vi "ExCenterStripStrNframe.vi"() -> ()   [LabVIEW 2010]
panel:
  in  "Number of frames to store":u32=1 min=1 step=1
  out "Strip":sgl[](graph)
  in  "Temperature":dbl=-10.0 format="%.2f"
  in  "Exposure":dbl min=0.0 step=0.001 format="%.3f"
  out "error out":errorcluster
  in  "error in (no error)":errorcluster
  # "ExCenterStripStrNframe:\nThis example selects the center strip of the CCD for the ROI and then \ncollects the data using circular buffers. It collects data until the number \nof frames are stored."
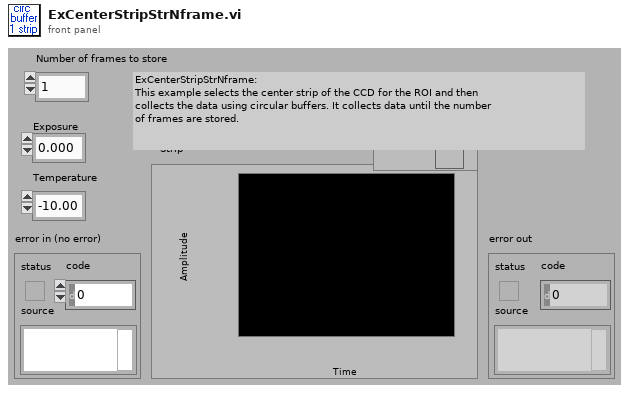
[diagram p1: front panel]
types:
  T1 = cluster{"Acquire / focus mode \n1 is Sync circualar buffers":i32, "Exposure":dbl, "Number of frames to store":u32, "Number of software\naccumulations":i32}
  T2 = cluster{"Camera Handle":u32, "Pulser Handle":u32, "File Handle":u32, "Display Handle":u32, "Image Handle":u32}
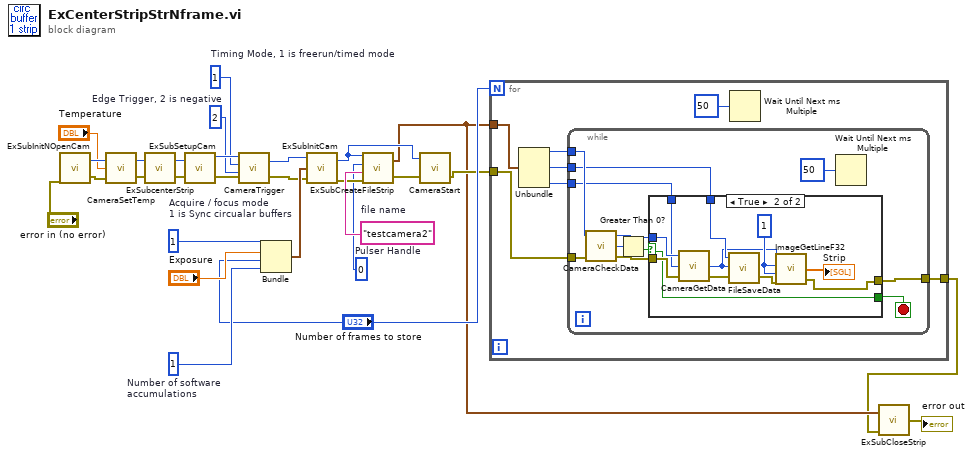
[diagram p0: block diagram]
diagram:
  w14 = 2  # Edge Trigger, 2 is negative
  w15 = 1  # Timing Mode, 1 is freerun/timed mode
  w21 = 0  # Pulser Handle
  w27 = 1  # Acquire / focus mode  1 is Sync circualar buffers
  w26 = 1  # Number of software accumulations
  w28 = "testcamera2"  # file name
  n1 = call "ExSubInitNOpenCam.vi"("error in (no error)"="error in (no error)") -> ("Camera Handle"=w7:u32, "error out"=w6:errorcluster)
  n2 = call <userlib>:"CameraSetTemp.vi"("error in (no error)"=w6, "Temperature"="Temperature", "Camera Handle"=w7) -> ("error out"=w8:errorcluster, "Camera Handle"=w9:u32)
  n3 = call "ExSubcenterStrip.vi"("error in (no error)"=w8, "Camera Handle"=w9) -> ("error out"=w11:errorcluster, "Camera Handle"=w10:u32)
  n4 = call "ExSubSetupCam.vi"("error in (no error)"=w11, "Camera Handle"=w10) -> ("error out"=w13:errorcluster, "Camera Handle"=w17:u32)
  n5 = call <userlib>:"CameraTrigger.vi"("error in"=w13, "Trigger Edge"=w14, "Timing Mode"=w15, "Camera Handle"=w17) -> ("error out"=w18:errorcluster, "Camera Handle"=w16:u32)
  n6 = Bundle("Acquire / focus mode \n1 is Sync circualar buffers"=w27, "Exposure"="Exposure", "Number of frames to store"="Number of frames to store", "Number of software\naccumulations"=w26) -> (w23:T1)  [unwired: 1 in]
  n7 = call "ExSubInitCam.vi"("error in (no error)"=w18, "Camera Information"=w23, "Camera Handle"=w16) -> ("error out"=w22:errorcluster, "Camera Handle"=w20:u32)
  n8 = call "ExSubCreateFileStrip.vi"("error in (no error)"=w22, "File and Display Name"=w28, "Pulser Handle"=w21, "Camera Handle"=w20) -> ("error out"=w12:errorcluster, "Handles Out"=w2:T2)
  n9 = call <userlib>:"CameraStart.vi"("error in"=w12, "Camera Handle"=w20) -> ("error out"=w3:errorcluster)  [unwired: 1 out]
  n10 = for {
    N: "Number of frames to store" -> [_]
    tunnel: w2 -> [w35]
    tunnel: w3 -> [w30]
    tunnel: [w29] -> w1
    n11 = Unbundle(w35) -> ("Camera Handle"=w34:u32, "File Handle"=w32:u32, "Image Handle"=w33:u32)  [unwired: 2 out]
    n12 = while {
      tunnel: [w41] -> w29
      tunnel: w34 -> [w39]
      tunnel: w33 -> [w38]
      tunnel: w32 -> [w37]
      tunnel: w30 -> [w36]
      stop <- w42 stop-if-true
      n13 = call <userlib>:"CameraCheckData.vi"("Camera Handle"=w39, "error in"=w36) -> ("Camera Handle"=w44:u32, "Number Of Frames Available"=w46:i32, "error out"=w43:errorcluster)
      n14 = Greater Than 0?(x=w46) -> (x > 0?=w45:bool)
      n15 = case shown="True" w45 {
        selector: w45 -> [w47 w57]
        tunnel: w44 -> [_ w59]
        tunnel: w43 -> [w48 w58]
        tunnel: [w47 w57] -> w42
        tunnel: [w48 w52] -> w41
        tunnel: w38 -> [_ w51]
        tunnel: w37 -> [_ w50]
        frame False {
        }
        frame True {
          w53 = 1
          n16 = call <userlib>:"CameraGetData.vi"("error in"=w58, "Data Handle"=w51, "Camera Handle"=w59) -> ("error out"=w56:errorcluster, "Data Handle"=w49:u32)  [unwired: 1 out]
          n17 = call <userlib>:"FileSaveData.vi"("error in"=w56, "Image Handle"=w49, "File Handle"=w50) -> ("error out"=w55:errorcluster)  [unwired: 1 out]
          n18 = call <userlib>:"ImageGetLineF32.vi"("error in"=w55, "Z Position"=w53, "Y Position"=w53, "Data Handle"=w49) -> ("error out"=w52:errorcluster, "Array F32"=→"Strip":sgl[])  [unwired: 1 out]
        }
      }
      n19 = Wait Until Next ms Multiple(millisecond multiple=u32 50) -> ()  [unwired: 1 out]
    }
    n20 = Wait Until Next ms Multiple(millisecond multiple=u32 50) -> ()  [unwired: 1 out]
  }
  n21 = call "ExSubCloseStrip.vi"("error in (no error)"=w1, "Handles In"=w2) -> ("error out"=→"error out":errorcluster)
